vi "Get_DistPart.vi"(8 "error in (no error)":errorcluster, 11 "Class in":refnum<class "IB_DistPart.lvclass">) -> (0 "error out":errorcluster, 2 "data":T1, 3 "Class out":refnum<class "IB_DistPart.lvclass">)   [LabVIEW 2020, in "IB_DistPart.lvclass"]
uses:
  <vilib>/AppBuilder/IB_Classes/DistPart/IB_DistPart.lvclass
  <vilib>/AppBuilder/IB_Classes/DistPart/IB_DistPart.lvclass/IB_DistPart.ctl
  <vilib>/AppBuilder/IB_Classes/DistPart/IB_DistPart.ctl
  <vilib>/AppBuilder/IB_Classes/DistPart/IB_FlavorInfo.ctl
  <vilib>/AppBuilder/IB_Classes/DistPart/IB_DistPartType.ctl
  <vilib>/AppBuilder/IB_Classes/SoftDependency/IB_SoftDependency.lvclass
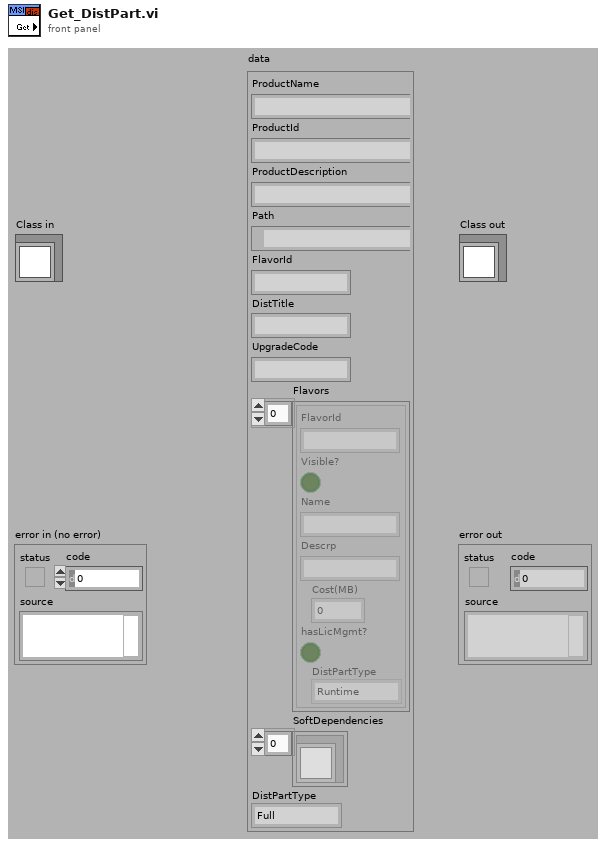
[diagram p1: front panel]
types:
  T1 = typedef "IB_DistPart.ctl" = cluster{"ProductName":string, "ProductId":string, "ProductDescription":string, "Path":path, "FlavorId":string, "DistTitle":string, "UpgradeCode":string, "Flavors":T2[], "SoftDependencies":refnum<class "IB_SoftDependency.lvclass">[], "DistPartType":T3}
  T2 = typedef "IB_FlavorInfo.ctl" = cluster{"FlavorId":string, "Visible?":bool, "Name":string, "Descrp":string, "Cost(MB)":i32, "hasLicMgmt?":bool, "DistPartType":T3}
  T3 = typedef "IB_DistPartType.ctl" = enum16{"Full", "Runtime"}
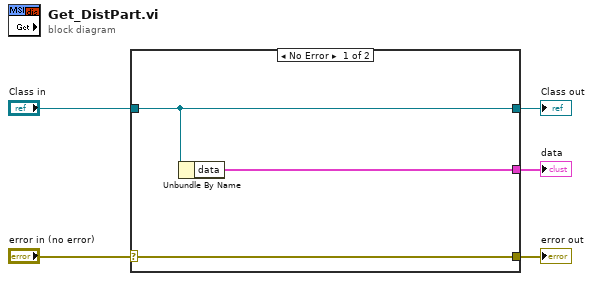
[diagram p0: block diagram]
diagram:
  n1 = case shown="No Error" "error in (no error)" {
    selector: "error in (no error)" -> [w8 w9]
    tunnel: [w8 w9] -> w4
    tunnel: [w7 w10] -> w2
    tunnel: "Class in" -> [w7 w10]
    tunnel: [w6 _] -> w1
    frame No Error {
      n2 = Unbundle By Name(w7) -> ("data"=w6:T1)
    }
    frame Error {
    }
  }
  "error out" <- w4
  "Class out" <- w2
  "data" <- w1
